vi "SSFG_simulated_Backup.vi"() -> ()   [LabVIEW 2014]
uses:
  <vilib>/measure/NI_MABase.lvlib
panel:
  in  "Sag Parameters":T1
  in  "stop":bool
  out "Final Waveform":waveform(dbl)(graph)
  out "Disturbance Mollifier":dbl[](graph)
  out "Pure Power Signal":waveform(dbl)(graph)
  in  "Power Signal Frequency (Hz)":dbl
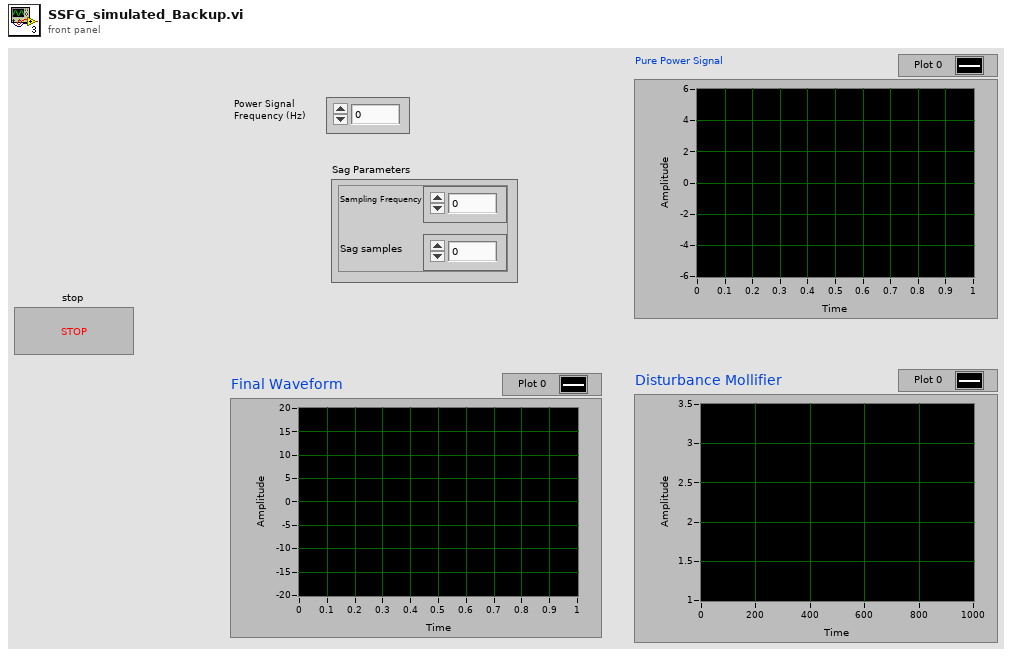
[diagram p1: front panel]
types:
  T1 = cluster{"Sampling Frequency":dbl, "Sag samples":dbl}
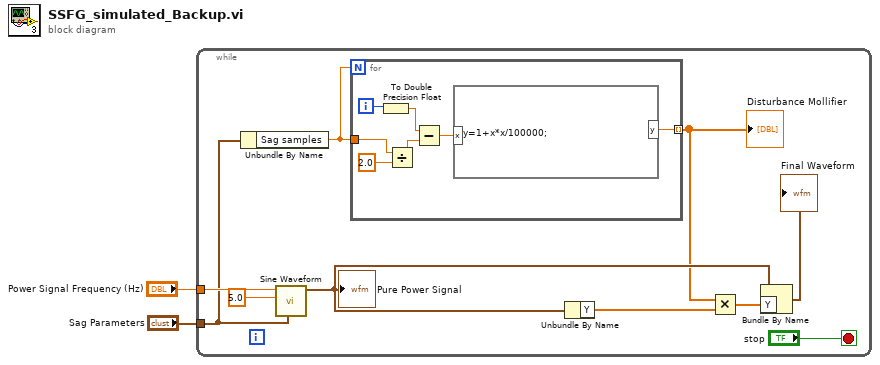
[diagram p0: block diagram]
diagram:
  n1 = while {
    tunnel: "Power Signal Frequency (Hz)" -> [w12]
    tunnel: "Sag Parameters" -> [w6]
    stop <- "stop" stop-if-true
    n2 = Unbundle By Name(w6) -> ("Sag samples"=w5:dbl)
    n3 = call <vilib>:"Sine Waveform.vi"("sampling info"=w6, "amplitude"=5.0, "frequency"=w12) -> ("signal out"=w8:waveform(dbl))  [unwired: 7 in, 1 out]
    "Pure Power Signal" <- w8
    n4 = for {
      N: w5 -> [_]
      tunnel: [w15] -> w4 mode=indexing
      tunnel: w5 -> [w13]
      i -> [w17]
      n5 = To Double Precision Float(number=w17) -> (double precision float=w14:dbl)
      n6 = Divide(x=w13, y=2.0) -> (x/y=w18:dbl)
      n7 = Subtract(x=w14, y=w18) -> (x-y=w16:dbl)
      n8 = formula code="y=1+x*x/100000;"("x"=w16) -> ("y"=w15:dbl)
    }
    "Disturbance Mollifier" <- w4
    n9 = Unbundle By Name(w8) -> ("Y"=w3:dbl[])
    n10 = Multiply(x=w4, y=w3) -> (x*y=w10:dbl[])
    n11 = Bundle By Name(cluster=w8, "Y"=w10) -> (→"Final Waveform":waveform(dbl))
  }
